vi "FL_Last_N_Samples.vi"(1 "BufferLengthSamples":u32=10000, 2 "InputArray":sgl[][](array[numeric])) -> (0 "OutputArray":sgl[][](array[numeric]))   [LabVIEW 2016]
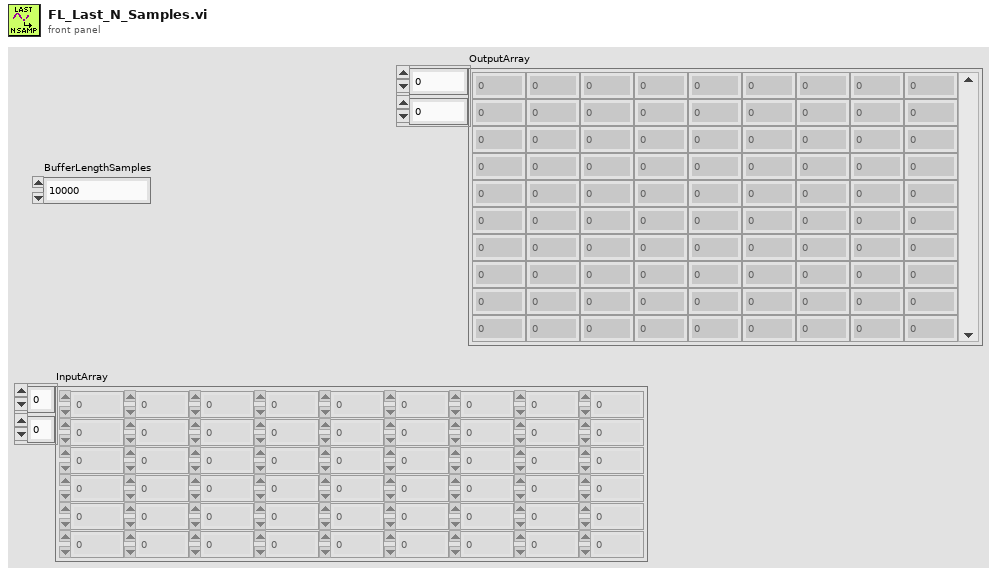
[diagram p1: front panel]
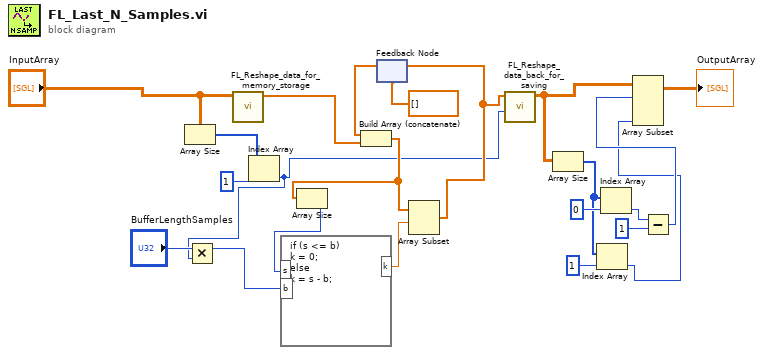
[diagram p0: block diagram]
diagram:
  n1 = Array Size(array="InputArray") -> (size(s)=w6:i32[])
  n2 = call "FL_Reshape_data_for_memory_storage.vi"("DEC SGL input"="InputArray") -> ("DEC SGL Output"=w14:sgl[])  [unwired: 10 in]
  n3 = Index Array(array=w6, index=1) -> (element=w3:i32)
  n4 = Multiply(x="BufferLengthSamples", y=w3) -> (x*y=w4:u32)
  n5 = feedback #1(sgl[] []) -> (w13:sgl[])
  n6 = Build Array (concatenate)(w13, w14) -> (w11:sgl[])
  n7 = Array Size(array=w11) -> (size(s)=w10:i32)
  n8 = formula code="if (s <= b)\nk = 0;\nelse\nk = s - b;"("s"=w10, "b"=w4) -> ("k"=w9:dbl)
  n9 = Array Subset(array=w11, index=w9) -> (w12:sgl[])  [unwired: 1 in]
  n10 = feedback-in #1(w12) -> ()
  n11 = call "FL_Reshape_data_back_for_saving.vi"("Read frame size"=w3, "DEC SGL input"=w12) -> ("DEC SGL Output"=w18:sgl[][])  [unwired: 9 in]
  n12 = Array Size(array=w18) -> (size(s)=w17:i32[])
  n13 = Index Array(array=w17, index=1) -> (element=w2:i32)
  n14 = Index Array(array=w17, index=0) -> (element=w20:i32)
  n15 = Subtract(x=w20, y=1) -> (x-y=w16:i32)
  n16 = Array Subset(array=w18, index (row)=w16, length (col)=w2) -> (→"OutputArray":sgl[][])  [unwired: 2 in]
